vi "beads_DAQ.vi"() -> ()   [LabVIEW 2014]
panel:
  in  "signal type":T1(ring)
  in  "Flash laser at \ndata start?":bool
  in  "Add small amp?":bool
  in  "Small amp freq (Hz)":dbl=10.0 format="%0.2p"
  in  "Small amp":dbl=1.0 format="%0.2p"
  out "P_cc [torr]":dbl format="%#_3g"
  out "P_pirani [torr]":dbl format="%#_3g"
  out "T_elec_rack [C]":dbl
  out "T_opt_table [C]":dbl
  in  "Read pressures?":bool
  in  "Read temps?":bool
  in  "Flash lamp\n settings:":T2={"Flash lamp?"=FALSE, "Number of cyles\nbetween flashes"=3, "# Pulses"=35, "Stop flashing \nbelow thresh?"=FALSE, "Stop threshold"=0.001, "Pulse voltage?"=FALSE, "Pulse length (ms)"=0.001, "Pulse amp (V)"=0.001}
  in  "Stage settings:":T3={"Set stage?"=FALSE, "start X (um)"=0.0, "stop X (um) "=0.0, "# X Steps"=1, "start Y (um)"=6.0, "stop Y (um) "=6.0, "# Y steps"=1, "start Z (um)"=4.0, "stop Z (um)"=4.0, "# Z steps "=1, "Sweep?"=FALSE, "Dir to sweep"=2, "Amplitude (um)"=4.0, "Frequency (Hz)"=3.7} {"Dir to sweep" items=["X", "Y", "Z"]}
  in  "Electrode settings:":T4={"DC volts (V):\n"=[0.0, 0.0, 0.0, 0.0, 0.0, 0.0, 0.0, 0.0], "Electrode to sweep:"=3, "start volt (V)"=1.5, "stop volt (V) "=1.5, "# V Steps"=1, "start freq (Hz)"=41.0, "stop freq (Hz) "=41.0, "# F steps"=1, "start DC (V)"=0.0, "stop DC (V)"=0.0, "# DC steps "=1, "Digitize electrode\ndrives?"=TRUE, "Sweep electrode?"=FALSE, "Add 0.5*V DC \noffset for amp?"=FALSE, "Use electrode \nconfig file?"=FALSE, "Path"=path "C:/GitHub/opt_lev/labview/DAQ_settings/electrode_sweep.txt", "Use arbitrary\nforce func?"=FALSE, "Voltage vs pos file"=path "C:/GitHub/opt_lev/labview/DAQ_settings/electrode_sweep.txt"}
  in  "DC supply settings:":T5
  in  "Synth settings:":T6={"start volt (V)"=1.0, "stop volt (V) "=1.0, "# V Steps"=1, "start freq (Hz)"=2000.0, "stop freq (Hz) "=2000.0, "# F steps"=1, "dc offset?"=FALSE, "start DC (V)"=0.5, "stop DC (V)"=0.5, "# DC steps "=1, "Set synth\n(HP33120A)?"=FALSE, "Use arbitrary\nwaveform?"=FALSE, "Arb waveform name:"=""}
  out "Waveform \nGraph":dbl[][](graph)
  out "Curr threshold":dbl
  in  "Number of Samples":i32=50000
  in  "Sample Rate [Hz]":dbl=5000.0
  out "Actual Sample \nRate":dbl=5000.0 format="%0.2f"
  in  "Delay between files [s]":dbl caption="Delay Time (s)"
  in  "Num files":i32=1
  in  "File base name":string="1_5mbar_nocool"
  in  "Directory path":path=path "C:/Data/20151026/bead1"
  # "Logging Settings"
  # "Environment"
  # "Flash Lamp Settings"
  # "0"
  # "1"
  # "2"
  # "3"
  # "4"
  # "5"
  # "6"
  # "7"
  # "Acquired Data"
  # "Timing Settings"
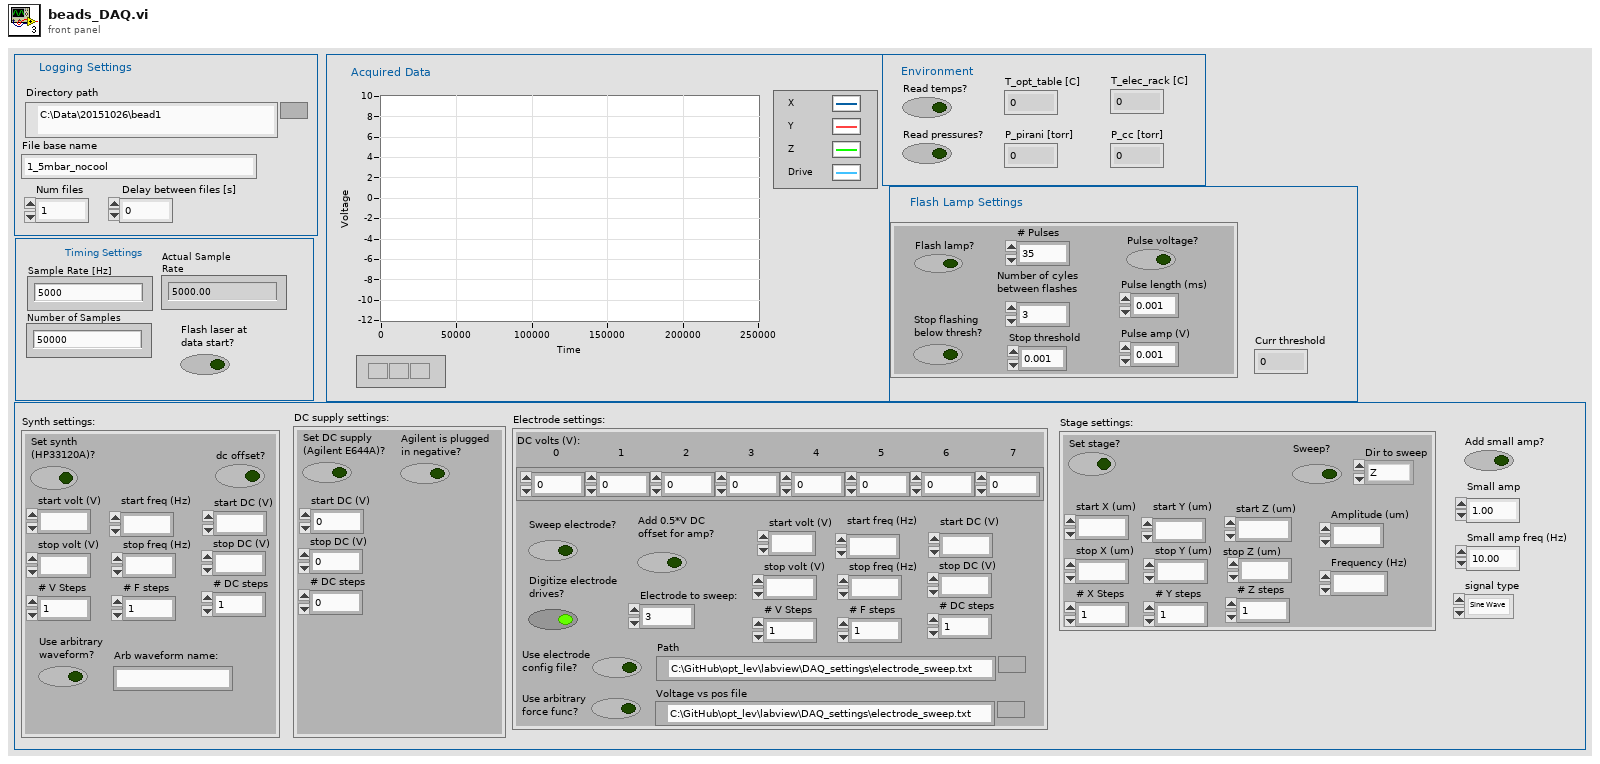
[diagram p1: front panel]
types:
  T1 = enum16{"Sine Wave", "Triangle Wave", "Square Wave", "Sawtooth Wave"}
  T2 = cluster{"Flash lamp?":bool, "Number of cyles\nbetween flashes":i32, "# Pulses":i32, "Stop flashing \nbelow thresh?":bool, "Stop threshold":dbl, "Pulse voltage?":bool, "Pulse length (ms)":dbl, "Pulse amp (V)":dbl}
  T3 = cluster{"Set stage?":bool, "start X (um)":ext, "stop X (um) ":ext, "# X Steps":i32, "start Y (um)":ext, "stop Y (um) ":ext, "# Y steps":i32, "start Z (um)":ext, "stop Z (um)":ext, "# Z steps ":i32, "Sweep?":bool, "Dir to sweep":u16, "Amplitude (um)":ext, "Frequency (Hz)":ext}
  T4 = cluster{"DC volts (V):\n":dbl[], "Electrode to sweep:":i32, "start volt (V)":ext, "stop volt (V) ":ext, "# V Steps":i32, "start freq (Hz)":ext, "stop freq (Hz) ":ext, "# F steps":i32, "start DC (V)":ext, "stop DC (V)":ext, "# DC steps ":i32, "Digitize electrode\ndrives?":bool, "Sweep electrode?":bool, "Add 0.5*V DC \noffset for amp?":bool, "Use electrode \nconfig file?":bool, "Path":path, "Use arbitrary\nforce func?":bool, "Voltage vs pos file":path}
  T5 = cluster{"start DC (V)":ext, "stop DC (V)":ext, "# DC steps ":i32, "Set DC supply\n(Agilent E644A)? ":bool, "Agilent is plugged \nin negative?":bool}
  T6 = cluster{"start volt (V)":ext, "stop volt (V) ":ext, "# V Steps":i32, "start freq (Hz)":ext, "stop freq (Hz) ":ext, "# F steps":i32, "dc offset?":bool, "start DC (V)":ext, "stop DC (V)":ext, "# DC steps ":i32, "Set synth\n(HP33120A)?":bool, "Use arbitrary\nwaveform?":bool, "Arb waveform name:":string}
  T7 = cluster{"Tot Synth Arr":dbl[], "Tot DC Arr":dbl[], "Tot Electrode Arr":dbl[], "Tot Stage Arr":dbl[]}[]
  T8 = cluster{"dup VISA session":refnum<visa-resource-name>, "error out":errorcluster, "task out":refnum<k21>, "error out":errorcluster}
  T9 = cluster{"Number of Samples":i32, "Sample Rate [Hz]":dbl, "Physical Channels (Position signals)":tag, "Physical Channel (drive signals)":tag, "Sample Clock Source":tag, "Physical Channel (drive signals)":tag}
  T10 = cluster{"Output channel (for flashing)":tag, i32, "path out":path, "Flash lamp\n settings:":cluster{"Flash lamp?":bool, "Number of cyles\nbetween flashes":i32, "# Pulses":i32, "Stop flashing \nbelow thresh?":bool, "Stop threshold":dbl, "Pulse voltage?":bool, "Pulse length (ms)":dbl, "Pulse amp (V)":dbl}}
  T11 = cluster{"dup VISA session":refnum<visa-resource-name>, "error out":errorcluster, "Agilent is \nplugged in \nnegative?":bool, "electrodes task":refnum<k21>, "electrodes task error":errorcluster, "Set synth":bool, "Set DC":bool}
  T12 = cluster{"data task":refnum<k21>, "data task error":errorcluster, "drive task":refnum<k21>, "drive task error":errorcluster, "trigger task":refnum<k21>, "trigger task error":errorcluster, "sample rate":dbl}
  T13 = cluster{"task out":refnum<k21>, "error out":errorcluster, "task out":refnum<k21>, "error out":errorcluster, "trigger task":refnum<k21>, "trigger task error":errorcluster}
  T14 = cluster{"data task":refnum<k21>, "data task error":errorcluster, "drive task":refnum<k21>, "drive task error":errorcluster, "trigger task":refnum<k21>, "trigger task error":errorcluster}
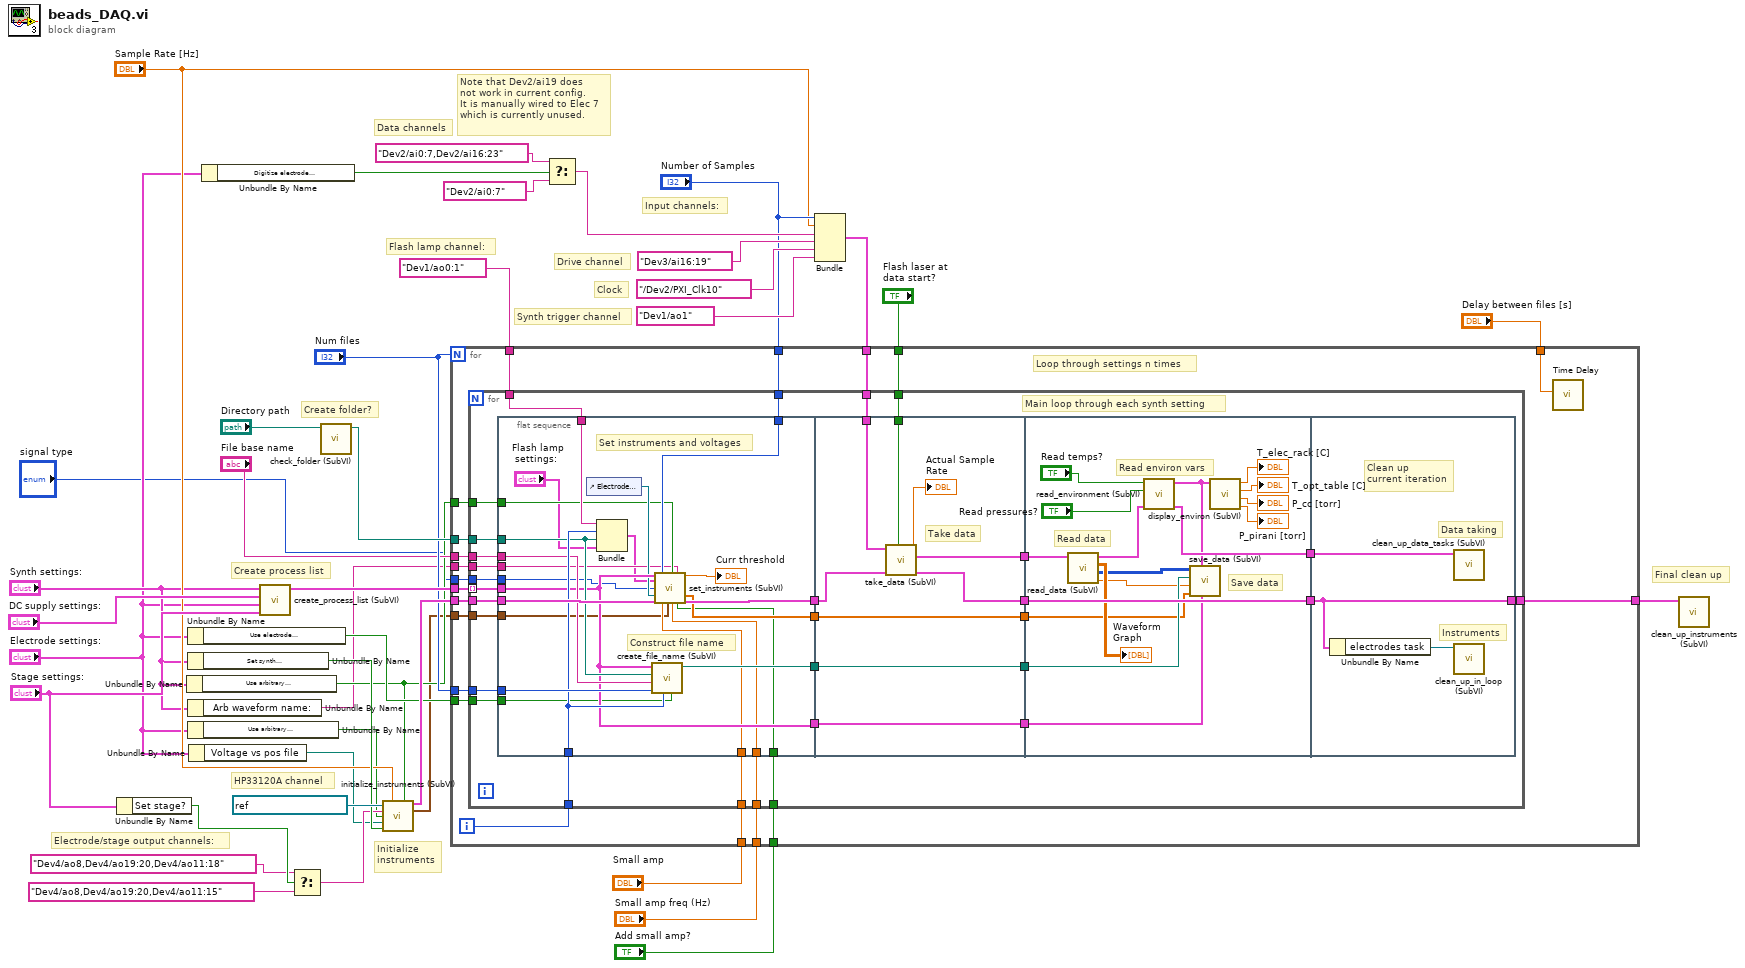
[diagram p0: block diagram]
diagram:
  # "Note that Dev2/ai19 does\nnot work in current config.\nIt is manually wired to Elec 7\nwhich is currently unused."
  # "Clock"
  # "Drive channel"
  # "Synth trigger channel"
  # "Data channels"
  # "Initialize\ninstruments"
  # "Electrode/stage output channels:"
  # "HP33120A channel"
  # "Flash lamp channel:"
  # "Create process list"
  # "Final clean up"
  # "Input channels:"
  # "Create folder?"
  n1 = Unbundle By Name("Stage settings:") -> ("Set stage?"=w19:bool)
  n2 = Unbundle By Name("Synth settings:") -> ("Use arbitrary\nwaveform?"=w10:bool)
  n3 = Unbundle By Name("Electrode settings:") -> ("Use electrode \nconfig file?"=w14:bool)
  n4 = Unbundle By Name("Synth settings:") -> ("Set synth\n(HP33120A)?"=w35:bool)
  n5 = Unbundle By Name("Synth settings:") -> ("Arb waveform name:"=w9:string)
  n6 = Unbundle By Name("Electrode settings:") -> ("Use arbitrary\nforce func?"=w6:bool)
  n7 = Unbundle By Name("Electrode settings:") -> ("Voltage vs pos file"=w5:path)
  n8 = Unbundle By Name("Electrode settings:") -> ("Digitize electrode\ndrives?"=w25:bool)
  n9 = call "create_process_list (SubVI).vi"("Synth settings:"="Synth settings:", "DC supply settings:"="DC supply settings:", "Electrode settings:"="Electrode settings:", "Stage settings:"="Stage settings:") -> ("Process list"=w38:T7)  [unwired: 5 in]
  n10 = Select(t=tag "Dev4/ao8,Dev4/ao19:20,Dev4/ao11:18" ("Output channel (for flashing)"), s=w19, f=tag "Dev4/ao8,Dev4/ao19:20,Dev4/ao11:15" ("Output channel (for flashing)")) -> (s? t:f=w17:tag)
  n11 = call "check_folder (SubVI).vi"("path in"="Directory path") -> ("path out"=w37:path)  [unwired: 10 in]
  n12 = call "initialize_instruments (SubVI).vi"("VISA Refnum in"=refnum<visa-resource-name> "GPIB0::10::INSTR" ("VISA session"), "Sample rate"="Sample Rate [Hz]", "trig_wfm"=w10, "Electrode outupt channels"=w17, "make volt file"=w6, "volt file path"=w5, "Use synth?"=w35) -> ("instrument config"=w34:T8, "Volt vs pos array"=w4:cluster{dbl, dbl}[])  [unwired: 7 in]
  n13 = Select(t=tag "Dev2/ai0:7,Dev2/ai16:23" ("Physical Channels (Position signals)"), s=w25, f=tag "Dev2/ai0:7" ("Physical Channels (Position signals)")) -> (s? t:f=w22:tag)
  n14 = Bundle("Number of Samples"="Number of Samples", "Sample Rate [Hz]"="Sample Rate [Hz]", "Physical Channels (Position signals)"=w22, "Physical Channel (drive signals)"=tag "Dev3/ai16:19", "Sample Clock Source"=tag "/Dev2/PXI_Clk10", "Physical Channel (drive signals)"=tag "Dev1/ao1") -> (w28:T9)  [unwired: 1 in]
  n15 = for {
    N: "Num files" -> [_]
    tunnel: "Delay between files [s]" -> [w60]
    tunnel: w38 -> [w59]
    tunnel: tag "Dev1/ao0:1" ("Output channel (for flashing)") -> [w58]
    tunnel: w37 -> [w56]
    tunnel: w34 -> [w55]
    tunnel: "Num files" -> [w54]
    tunnel: "File base name" -> [w53]
    tunnel: w28 -> [w52]
    tunnel: [w51] -> w27
    tunnel: "Number of Samples" -> [w50]
    tunnel: w14 -> [w49]
    tunnel: "Small amp" -> [w48]
    tunnel: "Small amp freq (Hz)" -> [w47]
    tunnel: "Add small amp?" -> [w46]
    tunnel: w10 -> [w45]
    tunnel: w9 -> [w44]
    tunnel: w4 -> [w43]
    tunnel: "Flash laser at \ndata start?" -> [w42]
    tunnel: "signal type" -> [w41]
    i -> [w57]
    # "Loop through settings n times"
    n16 = for {
      tunnel: w59 -> [w90] mode=indexing
      tunnel: w58 -> [w89]
      tunnel: w57 -> [w88]
      tunnel: w56 -> [w87]
      tunnel: w55 -> [w86]
      tunnel: w54 -> [w82]
      tunnel: w53 -> [w81]
      tunnel: w52 -> [w80]
      tunnel: [w75] -> w51
      tunnel: w50 -> [w70]
      tunnel: w49 -> [w69]
      tunnel: w48 -> [w68]
      tunnel: w47 -> [w67]
      tunnel: w46 -> [w66]
      tunnel: w45 -> [w65]
      tunnel: w44 -> [w64]
      tunnel: w43 -> [w63]
      tunnel: w42 -> [w62]
      tunnel: w41 -> [w61]
      # "Main loop through each synth setting"
      n17 = flat-sequence {
        tunnel: w90 -> [w104]
        tunnel: w89 -> [w113]
        tunnel: w88 -> [w108]
        tunnel: w87 -> [w107]
        tunnel: w86 -> [w111]
        tunnel: [w110] -> w83
        tunnel: w82 -> [w109]
        tunnel: w81 -> [w106]
        tunnel: [w105] -> w77
        tunnel: [w104] -> w74
        tunnel: [w102] -> w72
        tunnel: w70 -> [w101]
        tunnel: w69 -> [w100]
        tunnel: w68 -> [w99]
        tunnel: w67 -> [w98]
        tunnel: w66 -> [w97]
        tunnel: w65 -> [w96]
        tunnel: w64 -> [w95]
        tunnel: w63 -> [w94]
        tunnel: w61 -> [w91]
        tunnel: [w116] -> w84
        tunnel: w83 -> [w117]
        tunnel: w80 -> [w121]
        tunnel: [w119] -> w79
        tunnel: [w120] -> w78
        tunnel: w77 -> [w120]
        tunnel: w74 -> [w118]
        tunnel: [w118] -> w73
        tunnel: w72 -> [w115]
        tunnel: [w115] -> w71
        tunnel: w62 -> [w114]
        tunnel: [w139] -> w85
        tunnel: w84 -> [w139]
        tunnel: w79 -> [w138]
        tunnel: w78 -> [w135]
        tunnel: [w126] -> w76
        tunnel: w73 -> [w124]
        tunnel: w71 -> [w123]
        tunnel: w85 -> [w141]
        tunnel: w76 -> [w140]
        tunnel: [w141] -> w75
        frame #0 {
          # "Set instruments and voltages"
          # "Construct file name"
          n18 = control-ref of="Electrode settings:"() -> (w103:refnum<vi>)
          n19 = Bundle("Output channel (for flashing)"=w113, w108, "path out"=w107, "Flash lamp\n settings:"="Flash lamp\n settings:") -> (w93:T10)  [unwired: 1 in]
          n20 = call "create_file_name (SubVI).vi"("Use electrode config?"=w100, "file_idx"=w108, "num files"=w109, "base name"=w106, "Path"=w107, "Cluster"=w104) -> ("out path"=w105:path)  [unwired: 5 in]
          n21 = call "set_instruments (SubVI).vi"("Process list"=w104, "Flash lamp settings:"=w93, "signal type"=w91, "electrodes reference"=w103, "instrument config"=w111, "Num samples"=w101, "small amp"=w99, "Volt vs pos array"=w94, "wfm?"=w96, "small amp freq"=w98, "User Def. Wfm Name"=w95, "Add small amp?"=w97) -> ("Curr threshold"=→"Curr threshold":dbl, "DC volts arr"=w102:dbl[], "instrum out"=w110:T11)  [unwired: 5 in]
        }
        frame #1 {
          # "Take data"
          n22 = call "take_data (SubVI).vi"("trig?"=w114, "instrum in"=w117, "channel settings"=w121) -> ("instrum out"=w116:T11, "data tasks"=w119:T12, "Actual Sample Rate"=→"Actual Sample \nRate":dbl)  [unwired: 6 in]
        }
        frame #2 {
          # "Read environ vars"
          # "Read data"
          # "Save data"
          n23 = call "read_data (SubVI).vi"("data tasks"=w138) -> ("sample rate"=w134:dbl, "Rescaled data"=w136:i16[][], "Output data"=→"Waveform \nGraph":dbl[][], "output data tasks"=w127:T13)  [unwired: 7 in]
          n24 = call "read_environment (SubVI).vi"("data tasks"=w127, "Read pressures?"="Read pressures?", "Read temps?"="Read temps?") -> ("data tasks out"=w126:T14, "environ cluster"=w125:cluster{dbl[], dbl[]})  [unwired: 7 in]
          n25 = call "save_data (SubVI).vi"("Process list"=w124, "environ cluster"=w125, "DC volts arr"=w123, "Sample rate"=w134, "Filename"=w135, "data"=w136) -> ()  [unwired: 6 in]
          n26 = call "display_environ (SubVI).vi"("environ cluster"=w125) -> ("P_pirani"=→"P_pirani [torr]":dbl, "P_cc"=→"P_cc [torr]":dbl, "T_opt_table"=→"T_opt_table [C]":dbl, "T_elec_rack"=→"T_elec_rack [C]":dbl)  [unwired: 7 in]
        }
        frame #3 {
          # "Instruments"
          # "Data taking"
          # "Clean up\ncurrent iteration"
          n27 = Unbundle By Name(w141) -> ("electrodes task"=w142:refnum<k21>)
          n28 = call "clean_up_data_tasks (SubVI).vi"("data tasks"=w140) -> ()  [unwired: 11 in]
          n29 = call "clean_up_in_loop (SubVI).vi"("Refnum in"=w142) -> ()  [unwired: 10 in, 1 out]
        }
      }
    }
    n30 = call "Time Delay"("Delay Time (s)"=w60) -> ()  [unwired: 10 in, 1 out]
  }
  n31 = call "clean_up_instruments (SubVI).vi"("instrum out"=w27) -> ()  [unwired: 11 in]
